vi "Unflatten String 2D.vi"(11 "Tag value":string) -> (3 "String Array 2D":string[][](array[string]))   [LabVIEW 2020, in "NI_VIAn_XML Parsing.lvlib"]
uses:
  <vilib>/addons/analyzer/XML Parsing/NI_VIAn_XML Parsing.lvlib
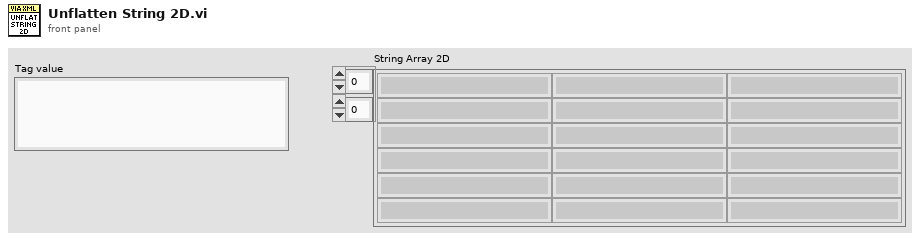
[diagram p1: front panel]
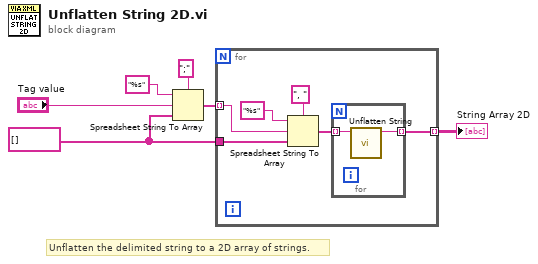
[diagram p0: block diagram]
diagram:
  w3 = string[] []
  # "Unflatten the delimited string to a 2D array of strings."
  n1 = Spreadsheet String To Array(delimiter (Tab)=";", format string="%s", spreadsheet string="Tag value", array type (2D Dbl)=w3) -> (array=w1:string[])
  n2 = for {
    tunnel: [w9] -> w6 mode=indexing
    tunnel: w3 -> [w8]
    tunnel: w1 -> [w7] mode=indexing
    n3 = Spreadsheet String To Array(delimiter (Tab)=", ", format string="%s", spreadsheet string=w7, array type (2D Dbl)=w8) -> (array=w10:string[])
    n4 = for {
      tunnel: w10 -> [w14] mode=indexing
      tunnel: [w13] -> w9 mode=indexing
      n5 = call <vilib>:"Unflatten String.vi"("Tag value"=w14) -> ("String"=w13:string)  [unwired: 10 in]
    }
  }
  "String Array 2D" <- w6
